vi "Parse InvertedSection.vi"(8 "Error In":errorcluster) -> (0 "Error Out":errorcluster)   [LabVIEW 2018, in "Tests.lvlib" / "Parser.lvlib"]
uses:
  Parser.lvlib
  src/Toolkit/Tokens/InvertedSection/InvertedSection.lvclass
  src/Toolkit/Tokens/Keyable/API/Keyable.lvclass/Keyable.ctl
  src/Toolkit/Tokens/Keyable/API/Read Key.vi
  src/Toolkit/Readers/String/String.lvclass
  D:/Users/cfield/Code/Field R&D Services/Mustache/trunk/src/Toolkit/Readers/Abstract/Abstract.lvclass
  <vilib>/Utility/LVClass/Get LV Class Name.vi
  src/Toolkit/Tokens/Keyable/API/Keyable.lvclass
  <vilib>/addons/_JKI Toolkits/Caraya/classes/Test/Test.lvclass
  <vilib>/addons/_JKI Toolkits/Caraya/classes/Assert/Assert.lvclass
  Tests.lvlib
  src/Toolkit/Toolkit.lvlib
  src/Toolkit/Tokens/Abstract/Abstract.lvclass
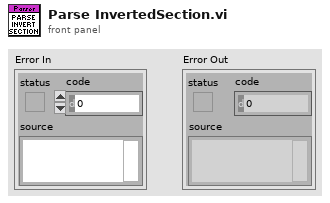
[diagram p1: front panel]
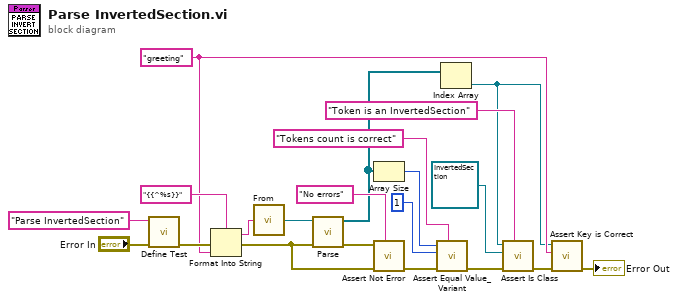
[diagram p0: block diagram]
diagram:
  w5 = "greeting"
  n1 = call <vilib>:"Define Test.vi"("error in (no error)"="Error In", "Label (VI Title)"="Parse InvertedSection") -> ("error out"=w18:errorcluster)  [unwired: 9 in]
  n2 = Format Into String(format string="{{^%s}}", error in=w18, w5) -> (resulting string=w7:string, error out=w2:errorcluster)  [unwired: 1 in]
  n3 = call "From.vi"("String"=w7) -> ("String"=w1:refnum<class "String.lvclass">)
  n4 = call "Parse.vi"("Error In"=w2, "Reader"=w1) -> ("Error Out"=w19:errorcluster, "Tokens"=w12:refnum<class "Abstract.lvclass">[])  [unwired: 8 in]
  n5 = Array Size(array=w12) -> (size(s)=w14:i32)
  n6 = call <vilib>:"Assert Not Error.vi"("Label"="No errors", "error in (no error)"=w2, "Not Error?"=w19) -> ("error out"=w16:errorcluster)  [unwired: 8 in]
  n7 = call <vilib>:"Assert Equal Value_Variant.vi"("Label"="Tokens count is correct", "error in (no error)"=w16, "Y"=1 ("size(s)"), "X"=w14) -> ("error out"=w11:errorcluster)  [unwired: 7 in]
  n8 = Index Array(array=w12) -> (element=w4:refnum<class "Abstract.lvclass">)  [unwired: 1 in]
  n9 = call "Assert Is Class.vi"("Label"="Token is an InvertedSection", "Error In"=w11, "Expected"=refnum<class "InvertedSection.lvclass"> refnum ("Mustache.lvlib:Tokens.lvlib:InvertedSection.lvclass"), "Actual"=w4) -> ("Error Out"=w9:errorcluster)  [unwired: 7 in]
  n10 = call "Assert Key is Correct.vi"("Error In"=w9, "Expected"=w5, "Token"=w4) -> ("Error Out"=→"Error Out":errorcluster)  [unwired: 8 in]
